vi "Path Mode Matrix SLM.vi"() -> (4 "mode matrix path":path)   [LabVIEW 2014]
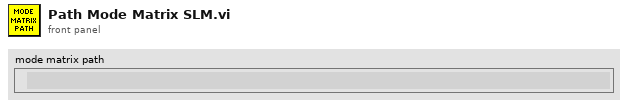
[diagram p1: front panel]
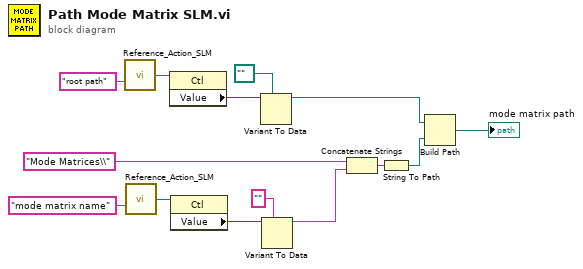
[diagram p0: block diagram]
diagram:
  n1 = call "Reference_Action_SLM.vi"("Control Name"="root path") -> ("Ref OUT"=w13:refnum<vi>)  [unwired: 12 in, 2 out]
  n2 = call "Reference_Action_SLM.vi"("Control Name"="mode matrix name") -> ("Ref OUT"=w7:refnum<vi>)  [unwired: 12 in, 2 out]
  n3 = property class="Ctl"(reference=w13) -> ("Value"=w12:variant)  [unwired: 1 in, 2 out]
  n4 = property class="Ctl"(reference=w7) -> ("Value"=w6:variant)  [unwired: 1 in, 2 out]
  n5 = Variant To Data(type=path "" ("Path"), Variant=w12) -> (data=w10:path)  [unwired: 1 in, 1 out]
  n6 = Variant To Data(type="", Variant=w6) -> (data=w1:string)  [unwired: 1 in, 1 out]
  n7 = Concatenate Strings("Mode Matrices\\" ("name or relative path"), w1) -> (w4:string)
  n8 = String To Path(string=w4) -> (path=w3:path)
  n9 = Build Path(base path=w10, name or relative path=w3) -> (appended path=→"mode matrix path":path)
